vi "SearchChannel.vi"(8 "error in":errorcluster, 10 "T560Channel.lvclass":refnum<class "T560Channel.lvclass">, 11 "T560Session in":refnum<class "T560Session.lvclass">) -> (0 "error out":errorcluster, 1 "Index":i32, 2 "T560Object.lvclass":refnum<class "T560Channel.lvclass">, 3 "T560Session out":refnum<class "T560Session.lvclass">)   [LabVIEW 2013, in "T560Session.lvclass"]
uses:
  T560Session.lvclass
  T560Channel.lvclass
  T560Session.lvclass/T560Session.ctl
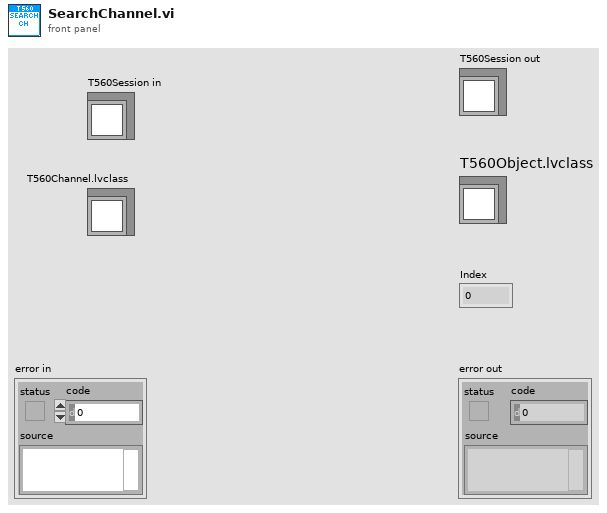
[diagram p1: front panel]
types:
  T1 = typedef "T560Channel.lvclass/ChannelName.ctl" = enum16{"Null", "A", "B", "C", "D", "Trigger"}
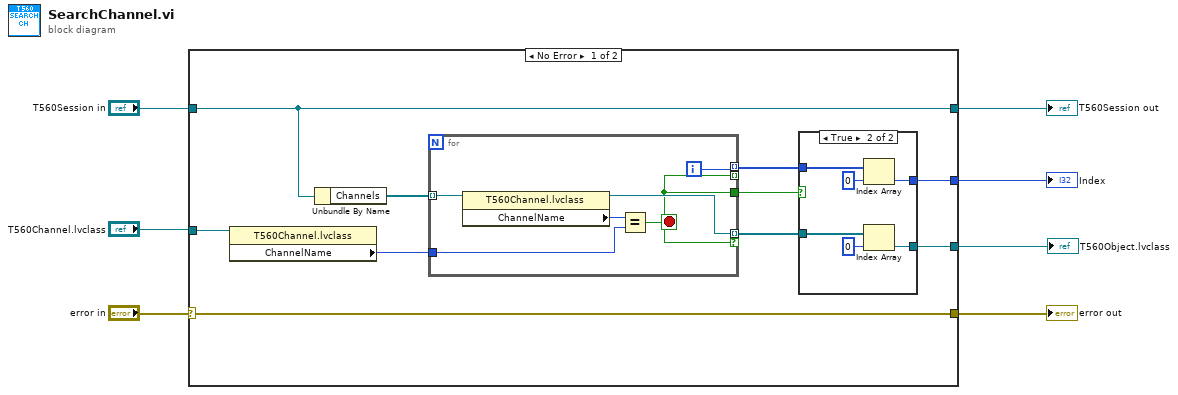
[diagram p0: block diagram]
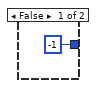
[diagram p2: hidden frame]
diagram:
  n1 = case shown="No Error" "error in" {
    selector: "error in" -> [w10 w32]
    tunnel: [w10 w32] -> w7
    tunnel: [w17 w31] -> w5
    tunnel: "T560Session in" -> [w17 w31]
    tunnel: [w14 _] -> w4
    tunnel: "T560Channel.lvclass" -> [w12 _]
    tunnel: [w8 _] -> w1
    frame No Error {
      n2 = property class="T560Channel.lvclass"(reference=w12) -> ("ChannelName"=w11:T1)  [unwired: 1 in, 2 out]
      n3 = Unbundle By Name(w17) -> ("Channels"=w16:refnum<class "T560Channel.lvclass">[])
      n4 = for {
        tunnel: w16 -> [w28] mode=indexing
        tunnel: w11 -> [w29]
        tunnel: [w30] -> w15 mode=indexing if=w25
        tunnel: [w25] -> _ mode=indexing
        tunnel: [w25] -> w13
        tunnel: [w26] -> w9 mode=indexing if=w25
        i -> [w30]
        stop <- w25 stop-if-true
        n5 = property class="T560Channel.lvclass"(reference=w28) -> (reference out=w26:refnum<class "T560Channel.lvclass">, "ChannelName"=w27:T1)  [unwired: 1 in, 1 out]
        n6 = Equal?(x=w27, y=w29) -> (x = y?=w25:bool)
      }
      n7 = case shown="True" w13 {
        tunnel: w15 -> [_ w24]
        tunnel: [-1 w22] -> w14
        tunnel: w9 -> [_ w21]
        tunnel: [_ w19] -> w8
        frame False {
        }
        frame True {
          n8 = Index Array(array=w24, index=0) -> (element=w22:i32)
          n9 = Index Array(array=w21, index=0) -> (element=w19:refnum<class "T560Channel.lvclass">)
        }
      }
    }
    frame Error {
    }
  }
  "error out" <- w7
  "T560Session out" <- w5
  "Index" <- w4
  "T560Object.lvclass" <- w1
